vi "Select Device.vi"(8 "error in (no error)":errorcluster, 10 "Device":refnum<class "Device.lvclass">, 11 "App in":refnum<class "App.lvclass">) -> (0 "error out":errorcluster, 3 "App out":refnum<class "App.lvclass">)   [LabVIEW 2020, in "PicoG-App.lvlib" / "App.lvclass"]
uses:
  App.lvclass
  Device/Device.lvclass
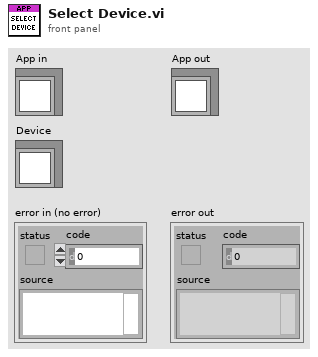
[diagram p1: front panel]
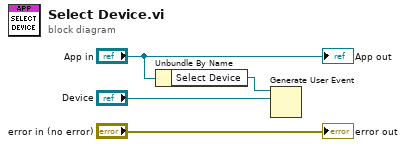
[diagram p0: block diagram]
diagram:
  n1 = Unbundle By Name("App in") -> ("Select Device"=w2:refnum<user-event>)
  n2 = Generate User Event(user event=w2, event data cluster="Device") -> ()  [unwired: 2 in, 2 out]
  "error out" <- "error in (no error)"
  "App out" <- "App in"
